vi "step_force_001.vi"(1 "Control Force in":dbl[unit], 2 "Current time":dbl[unit], 3 "time threshold":dbl[unit]) -> (0 "Control Force out":dbl[unit])   [LabVIEW 2019]
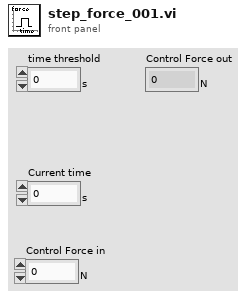
[diagram p1: front panel]
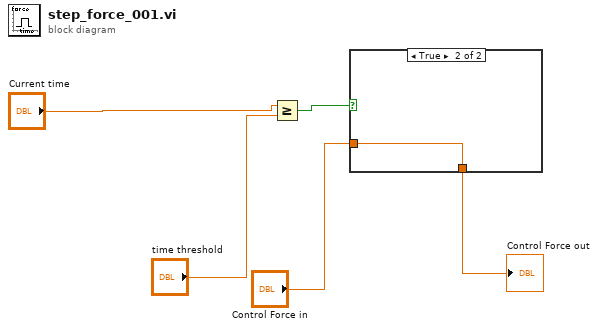
[diagram p0: block diagram]
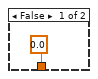
[diagram p2: hidden frame]
diagram:
  n1 = Greater Or Equal?(x="Current time", y="time threshold") -> (x >= y?=w1:bool)
  n2 = case shown="True" w1 {
    tunnel: "Control Force in" -> [_ w7]
    tunnel: [dbl[unit] 0.0 ("Control Force") w7] -> w3
    frame False {
    }
    frame True {
    }
  }
  "Control Force out" <- w3
